vi "列表初始化.vi"(11 "列表输入个数":i32) -> (3 "InitialData":string[][](array[string]))   [LabVIEW 2011]
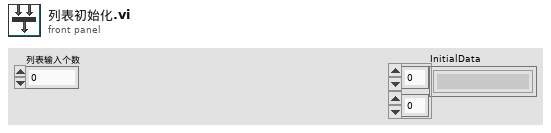
[diagram p1: front panel]
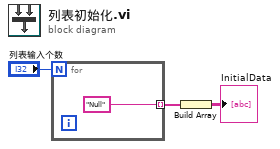
[diagram p0: block diagram]
diagram:
  n1 = for {
    N: "列表输入个数" -> [_]
    tunnel: ["Null"] -> w2 mode=indexing
  }
  n2 = Build Array(w2) -> (→"InitialData":string[][])
